vi "S_factor.vi"(10 "管内径[mm]":dbl, 11 "待测样品面积[mm^2]":dbl) -> (3 "S_factor":dbl)   [LabVIEW 2018]
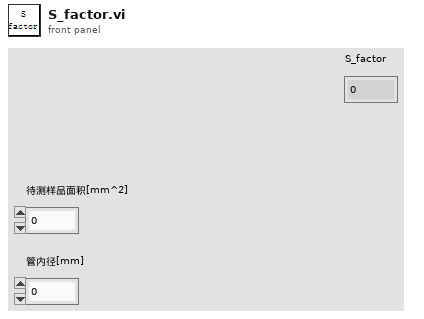
[diagram p1: front panel]
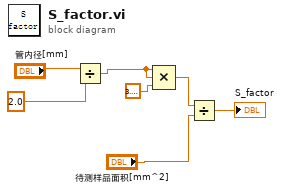
[diagram p0: block diagram]
diagram:
  n1 = Divide(x="管内径[mm]", y=2.0) -> (x/y=w6:dbl)
  n2 = Compound Arithmetic op=MULTIPLY(w6, w6, 3.141592653589793) -> (w3:dbl)
  n3 = Divide(x=w3, y="待测样品面积[mm^2]") -> (x/y=→"S_factor":dbl)
